vi "Change_Default_Destination.vi"(8 "error in (no error)":errorcluster, 9 "New default dest":string, 10 "Old default dest":string, 11 "IB_DestTree in":refnum<class "IB_Tree_Dest.lvclass">) -> (0 "error out":errorcluster, 3 "IB_DestTree out":refnum<class "IB_Tree_Dest.lvclass">)   [LabVIEW 2020, in "IB_Tree_Dest.lvclass"]
uses:
  <vilib>/AppBuilder/IB_Classes/Tree_Dest/IB_Tree_Dest.lvclass
  <vilib>/AppBuilder/IB_Classes/Tree_Dest/IB_Tree_Dest.lvclass/IB_Tree_Dest.ctl
  <vilib>/AppBuilder/IB_Classes/Tree/IB_Tree.lvclass
  <resource>/Framework/Providers/Builds/Installer/controls/IB_Tree_DefaultSymbols.ctl
  e:/builds/penguin/labview/branches/2020/dev/dist/vi.lib/AppBuilder/IB_Classes/Tree/IB_Tree.lvclass
  e:/builds/penguin/labview/branches/2020/dev/dist/vi.lib/AppBuilder/IB_Classes/Tree_Dest/IB_Tree_Dest.lvclass
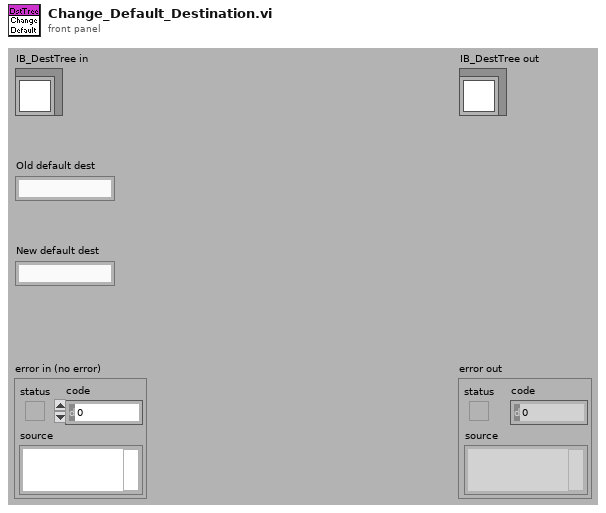
[diagram p1: front panel]
types:
  T1 = typedef "IB_Tree_DefaultSymbols.ctl" = enum16{"<unknown>", "closed folder", "open folder", "closed folder (default)", "open folder (default)", "closed sync folder", "open sync folder", "container folder", "my computer", "build specs", "exe", "dll", "source dist", "restful web service", ".net", "packed library", "c-generator", "target"}
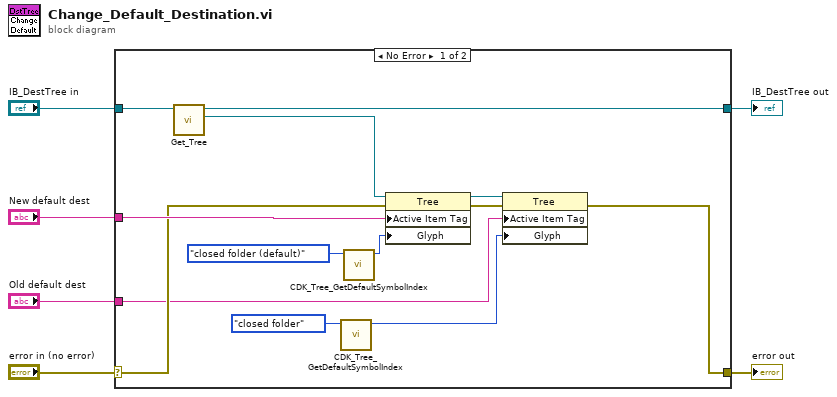
[diagram p0: block diagram]
diagram:
  n1 = case shown="No Error" "error in (no error)" {
    selector: "error in (no error)" -> [w9 w21]
    tunnel: [w8 w21] -> w5
    tunnel: [w18 w20] -> w3
    tunnel: "IB_DestTree in" -> [w19 w20]
    tunnel: "New default dest" -> [w10 _]
    tunnel: "Old default dest" -> [w7 _]
    frame No Error {
      n2 = call <vilib>:"Get_Tree.vi"("IB_Tree in"=w19) -> ("ctl"=w15:refnum<vi>, "IB_Tree out"=w18:refnum<class "IB_Tree_Dest.lvclass">)  [unwired: 8 in, 1 out]
      n3 = call <resource>:"CDK_Tree_GetDefaultSymbolIndex.vi"("default symbol"=IB_Tree_DefaultSymbols."closed folder") -> ("symbol index"=w13:i32)  [unwired: 9 in, 1 out]
      n4 = call <resource>:"CDK_Tree_GetDefaultSymbolIndex.vi"("default symbol"=IB_Tree_DefaultSymbols."closed folder (default)") -> ("symbol index"=w11:i32)  [unwired: 9 in, 1 out]
      n5 = property class="Tree"(reference=w15, error in=w9, "Active Item Tag"=w10, "Glyph"=w11) -> (reference out=w17:refnum<vi>, error out=w16:errorcluster)
      n6 = property class="Tree"(reference=w17, error in=w16, "Active Item Tag"=w7, "Glyph"=w13) -> (error out=w8:errorcluster)  [unwired: 1 out]
    }
    frame Error {
    }
  }
  "error out" <- w5
  "IB_DestTree out" <- w3
